vi "Write Input.vi"(8 "error in (no error)":errorcluster, 10 "Input":bool[](array[boolean]), 11 "TD4 in":refnum<class "TD4.lvclass">) -> (0 "error out":errorcluster, 3 "TD4 out":refnum<class "TD4.lvclass">)   [LabVIEW 2025, in "TD4.lvclass"]
uses:
  TD4.lvclass
  TD4.lvclass/TD4.ctl
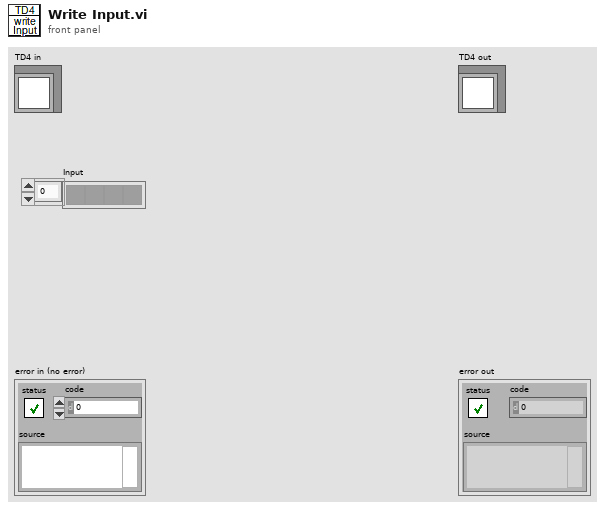
[diagram p1: front panel]
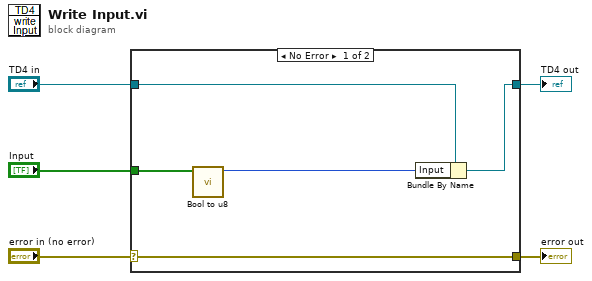
[diagram p0: block diagram]
diagram:
  n1 = case shown="No Error" "error in (no error)" {
    selector: "error in (no error)" -> [w10 w11]
    tunnel: [w10 w11] -> w4
    tunnel: [w8 w12] -> w2
    tunnel: "TD4 in" -> [w9 w12]
    tunnel: "Input" -> [w7 _]
    frame No Error {
      n2 = call "Bool to u8.vi"("Input"=w7) -> ("Output"=w6:u8)  [unwired: 10 in]
      n3 = Bundle By Name(cluster=w9, "Input"=w6) -> (w8:refnum<class "TD4.lvclass">)
    }
    frame Error {
    }
  }
  "error out" <- w4
  "TD4 out" <- w2
